vi "Exercise 10.vi"() -> (0 "Time":string, 1 "Date":string, 2 "User":string, 3 "Access":bool=TRUE)   [LabVIEW 2023]
panel:
  in  "Password":string
  in  "Login":string
  in  "Table":string[][](array[string])=[["admin", "labview"], ["user 1", "12345"], ["guest", ""]]
  in  "OK Button":bool
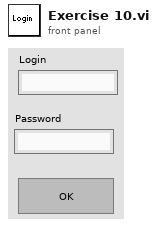
[diagram p1: front panel]
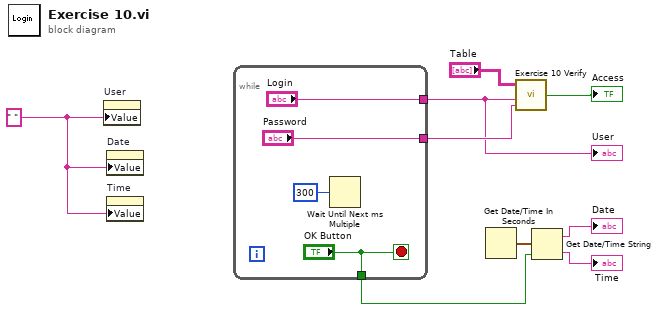
[diagram p0: block diagram]
diagram:
  w1 = " "
  n1 = property on="User" class="Str"("Value"=w1) -> ()  [unwired: 2 in, 2 out]
  n2 = property on="Date" class="Str"("Value"=w1) -> ()  [unwired: 2 in, 2 out]
  n3 = property on="Time" class="Str"("Value"=w1) -> ()  [unwired: 2 in, 2 out]
  n4 = while {
    tunnel: ["OK Button"] -> w8
    tunnel: ["Login"] -> w2
    tunnel: ["Password"] -> w4
    stop <- "OK Button" stop-if-true
    n5 = Wait Until Next ms Multiple(millisecond multiple=u32 300) -> ()  [unwired: 1 out]
  }
  "User" <- w2
  n6 = Get Date/Time In Seconds() -> (seconds since 1Jan1904=w9:timestamp)
  n7 = call "Exercise 10 Verify.vi"("Password"=w4, "Login"=w2, "Table"="Table") -> ("Access"=→"Access":bool)
  n8 = Get Date/Time String(seconds (now)=w9, want seconds? (F)=w8) -> (date string=→"Date":string, time string=→"Time":string)  [unwired: 1 in]
